vi "PI Close GPIB.vi"(0 "System no.":i32=1 min=1 max=4 step=1, 5 "error in":errorcluster) -> (14 "Was connected?":bool, 19 "error out":errorcluster)   [LabVIEW 2011]
doc: "This VI checks if the connection to the selected system is already open and, if it is, it closes this connection. \n\nValid for C-843, C-843.PM, C-844, C-865, E-710 (but must be present in Communication.llb for all other systems, too)"
uses:
  <userlib>/E710_GCS_LabVIEW/Low Level/Communication.llb/Global1.vi
panel:
  # "This vi checks if the connection to the selected system\nis already open and, if it is, it closes this connection."
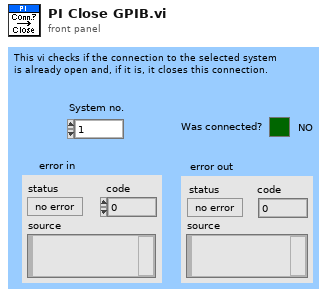
[diagram p1: front panel]
types:
  T1 = cluster{"DLL for Device":u16, "DLL Interface":u16, "Parameter":string}[]
  T2 = cluster{"RS232 Portnumber":u16, "Timeout":u32, "RS232 Baud rate":u32, "Interface":u16, "GPIB Bus":i32, "GPIB Address":i32, "GPIB Mode":i32}[]
  T3 = cluster{"RS232 Portnumber":u16, "Timeout":u32, "RS232 Baud rate":u32, "Interface":u16, "GPIB Bus":i32, "GPIB Address":i32, "GPIB Mode":i32}
  T4 = cluster{"DLL for Device":u16, "DLL Interface":u16, "Parameter":string}
  T5 = enum16{"C844_IsDLLAvailable", "C844_ConnectRS232", "C844_ConnectNIgpib", "C844_IsConnected", "C844_CloseConnection", "C844_GcsCommandset", "C844_GetError", "C844_GcsGetAnswerSize", "C844_GcsGetAnswer"}
  T6 = enum16{"C844_IsDLLAvailable", "C844_ConnectRS232", "C844_ConnectNIgpib", "C844_IsConnected", "C844_CloseConnection", "C844_GcsCommandset", "C844_GetError", "C844_GcsGetAnswerSize", "C844_GcsGetAnswer", "C843_IsDLLAvailable", "C843_Connect", "C843_IsConnected", "C843_CloseConnection", "C843_GcsCommandset", "C843_GetError", "C843_GcsGetAnswerSize", "C843_GcsGetAnswer", "E710_IsDLLAvailable", "E710_ConnectRS232", "E710_ConnectNIgpib", "E710_IsConnected", "E710_CloseConnection", "E710_GcsCommandset", "E710_GetError", "E710_GcsGetAnswerSize", "E710_GcsGetAnswer"}
  T7 = enum16{"C844_IsDLLAvailable", "C844_ConnectRS232", "C844_ConnectNIgpib", "C844_IsConnected", "C844_CloseConnection", "C844_GcsCommandset", "C844_GetError", "C844_GcsGetAnswerSize", "C844_GcsGetAnswer", "C843_IsDLLAvailable", "C843_Connect", "C843_IsConnected", "C843_CloseConnection", "C843_GcsCommandset", "C843_GetError", "C843_GcsGetAnswerSize", "C843_GcsGetAnswer", "E710_IsDLLAvailable", "E710_ConnectRS232", "E710_ConnectNIgpib", "E710_IsConnected", "E710_CloseConnection", "E710_GcsCommandset", "E710_GetError", "E710_GcsGetAnswerSize", "E710_GcsGetAnswer", "C843_PM_IsDLLAvailable", "C843_PM_Connect", "C843_PM_IsConnected", "C843_PM_CloseConnection", "C843_PM_GcsCommandset", "C843_PM_GetError", "C843_PM_GcsGetAnswerSize", "C843_PM_GcsGetAnswer", "C843_PM_GetCurrentBoardID"}
  T8 = enum16{"C844_IsDLLAvailable", "C844_ConnectRS232", "C844_ConnectNIgpib", "C844_IsConnected", "C844_CloseConnection", "C844_GcsCommandset", "C844_GetError", "C844_GcsGetAnswerSize", "C844_GcsGetAnswer", "C843_IsDLLAvailable", "C843_Connect", "C843_IsConnected", "C843_CloseConnection", "C843_GcsCommandset", "C843_GetError", "C843_GcsGetAnswerSize", "C843_GcsGetAnswer", "E710_IsDLLAvailable", "E710_ConnectRS232", "E710_ConnectNIgpib", "E710_IsConnected", "E710_CloseConnection", "E710_GcsCommandset", "E710_GetError", "E710_GcsGetAnswerSize", "E710_GcsGetAnswer", "C843_PM_IsDLLAvailable", "C843_PM_Connect", "C843_PM_IsConnected", "C843_PM_CloseConnection", "C843_PM_GcsCommandset", "C843_PM_GetError", "C843_PM_GcsGetAnswerSize", "C843_PM_GcsGetAnswer"}
  T9 = enum16{"C844_IsDLLAvailable", "C844_ConnectRS232", "C844_ConnectNIgpib", "C844_IsConnected", "C844_CloseConnection", "C844_GcsCommandset", "C844_GetError", "C844_GcsGetAnswerSize", "C844_GcsGetAnswer", "C843_IsDLLAvailable", "C843_Connect", "C843_IsConnected", "C843_CloseConnection", "C843_GcsCommandset", "C843_GetError", "C843_GcsGetAnswerSize", "C843_GcsGetAnswer", "E710_IsDLLAvailable", "E710_ConnectRS232", "E710_ConnectNIgpib", "E710_IsConnected", "E710_CloseConnection", "E710_GcsCommandset", "E710_GetError", "E710_GcsGetAnswerSize", "E710_GcsGetAnswer", "C843_PM_IsDLLAvailable", "C843_PM_Connect", "C843_PM_IsConnected", "C843_PM_CloseConnection", "C843_PM_GcsCommandset", "C843_PM_GetError", "C843_PM_GcsGetAnswerSize", "C843_PM_GcsGetAnswer", "C843_PM_GetCurrentBoardID", "C843_GetCurrentBoardID", "C865_IsDLLAvailable", "C865_ConnectRS232", "C865_IsConnected", "C865_CloseConnection", "C865_GcsCommandset", "C865_GetError", "C865_GcsGetAnswerSize", "C865_GcsGetAnswer", "C865_GetCurrentInterfaceID"}
  T10 = enum16{"C844_IsDLLAvailable", "C844_ConnectRS232", "C844_ConnectNIgpib", "C844_IsConnected", "C844_CloseConnection", "C844_GcsCommandset", "C844_GetError", "C844_GcsGetAnswerSize", "C844_GcsGetAnswer", "C843_IsDLLAvailable", "C843_Connect", "C843_IsConnected", "C843_CloseConnection", "C843_GcsCommandset", "C843_GetError", "C843_GcsGetAnswerSize", "C843_GcsGetAnswer", "E710_IsDLLAvailable", "E710_ConnectRS232", "E710_ConnectNIgpib", "E710_IsConnected", "E710_CloseConnection", "E710_GcsCommandset", "E710_GetError", "E710_GcsGetAnswerSize", "E710_GcsGetAnswer", "C843_PM_IsDLLAvailable", "C843_PM_Connect", "C843_PM_IsConnected", "C843_PM_CloseConnection", "C843_PM_GcsCommandset", "C843_PM_GetError", "C843_PM_GcsGetAnswerSize", "C843_PM_GcsGetAnswer", "C843_PM_GetCurrentBoardID", "C843_GetCurrentBoardID"}
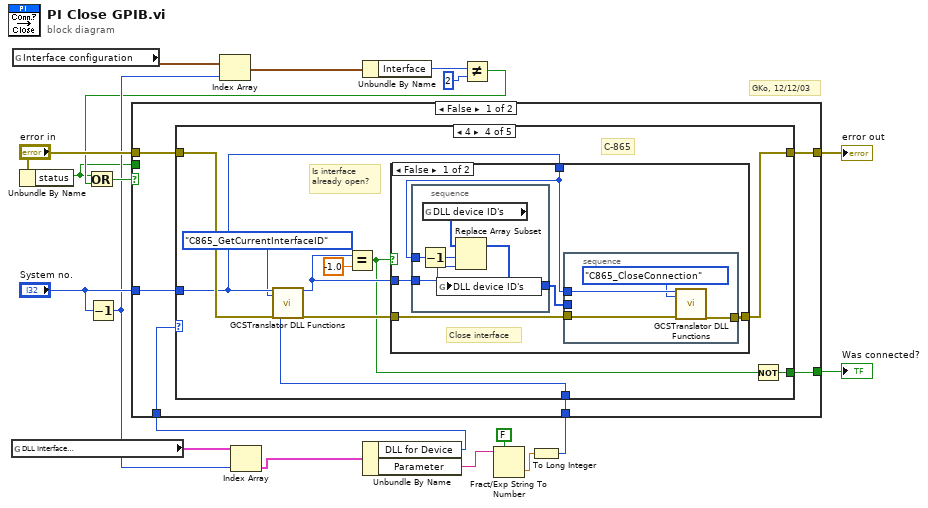
[diagram p0: block diagram]
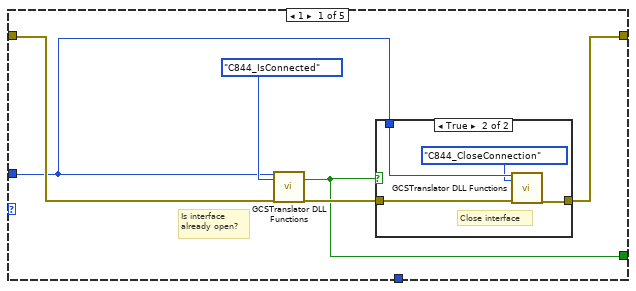
[diagram p2: hidden frame]
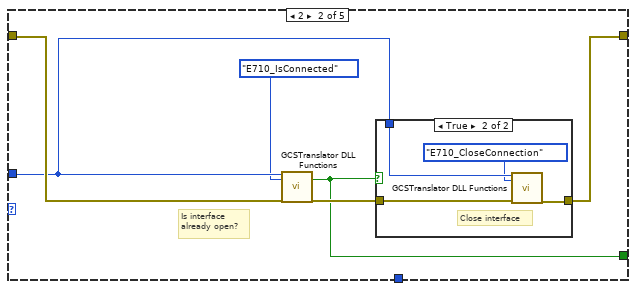
[diagram p4: hidden frame]
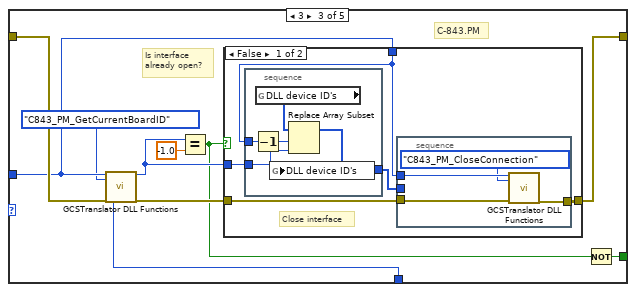
[diagram p6: hidden frame]
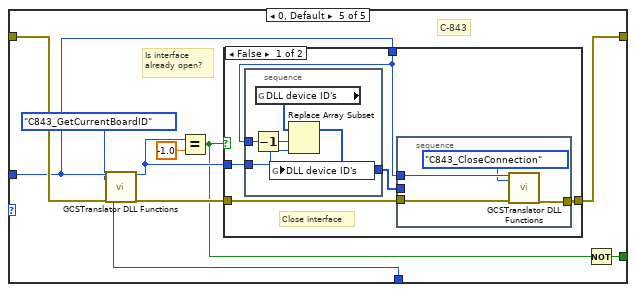
[diagram p9: hidden frame]
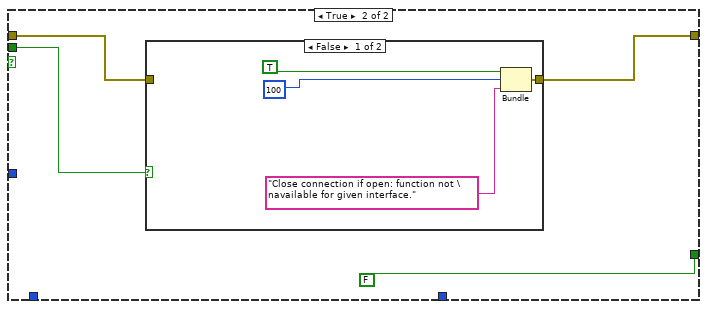
[diagram p11: hidden frame]
diagram:
  # "GKo, 12/12/03"
  n1 = global read "Global1.vi" "DLL Interface\nConfiguration"() -> (w16:T1)
  n2 = global read "Global1.vi" "Interface configuration"() -> (w13:T2)
  n3 = Unbundle By Name("error in") -> ("status"=w5:bool)
  n4 = Decrement(x="System no.") -> (x-1=w7:i32)
  n5 = Index Array(array=w13, index=w7) -> (element=w12:T3)
  n6 = Index Array(array=w16, index=w7) -> (element=w15:T4)
  n7 = Unbundle By Name(w12) -> ("Interface"=w11:u16)
  n8 = Unbundle By Name(w15) -> ("DLL for Device"=w14:u16, "Parameter"=w2:string)
  n9 = Not Equal?(x=w11, y=u16 2) -> (x != y?=w6:bool)
  n10 = Or(x=w5, y=w6) -> (x .or. y?=w9:bool)
  n11 = Fract/Exp String To Number(use system decimal point (T)=FALSE, string=w2) -> (number=w3:dbl)  [unwired: 2 in, 1 out]
  n12 = To Long Integer(number=w3) -> (32bit integer=w1:i32)
  n13 = case shown="False" w9 {
    tunnel: "System no." -> [w23 _]
    tunnel: "error in" -> [w25 w125]
    tunnel: [w24 w124] -> w18
    tunnel: [w22 FALSE ("Boolean output")] -> w17
    tunnel: w14 -> [w21 _]
    tunnel: w5 -> [_ w123]
    tunnel: w1 -> [w20 _]
    frame False {
      n14 = case shown="4" w21 {
        tunnel: w25 -> [w29 w41 w56 w81 w106]
        tunnel: [w28 w40 w55 w80 w105] -> w24
        tunnel: w23 -> [w27 w39 w54 w79 w104]
        tunnel: [w26 w38 w52 w77 w102] -> w22
        tunnel: w20 -> [_ _ w49 w74 w99]
        frame 1 {
          # "Is interface\nalready open?"
          n15 = call <userlib>:"GCSTranslator DLL Functions.vi"("System no."=w27, "Function"=T5."C844_IsConnected", "error in"=w29) -> ("Boolean output"=w26:bool, "error out"=w31:errorcluster)  [unwired: 12 in, 3 out]
          n16 = case shown="True" w26 {
            tunnel: w31 -> [w32 w36]
            tunnel: [w32 w35] -> w28
            tunnel: w27 -> [_ w34]
            frame False {
            }
            frame True {
              # "Close interface"
              n17 = call <userlib>:"GCSTranslator DLL Functions.vi"("System no."=w34, "Function"=T5."C844_CloseConnection", "error in"=w36) -> ("error out"=w35:errorcluster)  [unwired: 12 in, 4 out]
            }
          }
        }
        frame 2 {
          # "Is interface\nalready open?"
          n18 = call <userlib>:"GCSTranslator DLL Functions.vi"("System no."=w39, "Function"=T6."E710_IsConnected", "error in"=w41) -> ("Boolean output"=w38:bool, "error out"=w42:errorcluster)  [unwired: 12 in, 3 out]
          n19 = case shown="True" w38 {
            tunnel: w42 -> [w43 w47]
            tunnel: [w43 w46] -> w40
            tunnel: w39 -> [_ w45]
            frame False {
            }
            frame True {
              # "Close interface"
              n20 = call <userlib>:"GCSTranslator DLL Functions.vi"("System no."=w45, "Function"=T6."E710_CloseConnection", "error in"=w47) -> ("error out"=w46:errorcluster)  [unwired: 12 in, 4 out]
            }
          }
        }
        frame 3 {
          # "C-843.PM"
          # "Is interface\nalready open?"
          n21 = call <userlib>:"GCSTranslator DLL Functions.vi"("System no."=w54, "Function"=T7."C843_PM_GetCurrentBoardID", "error in"=w56, "Numerical input"=w49) -> ("DLL I32 Return value"=w51:i32, "error out"=w57:errorcluster)  [unwired: 11 in, 3 out]
          n22 = Equal?(x=w51, y=-1.0) -> (x = y?=w50:bool)
          n23 = case shown="False" w50 {
            tunnel: w57 -> [w62 w72]
            tunnel: [w61 w72] -> w55
            tunnel: w54 -> [w59 _]
            tunnel: w51 -> [w58 _]
            frame False {
              # "Close interface"
              n24 = stacked-sequence {
                tunnel: [w67] -> w60
                tunnel: w59 -> [w69]
                tunnel: w58 -> [w68]
                frame #0 {
                  n25 = Decrement(x=w69) -> (x-1=w70:i32)
                  n26 = global read "Global1.vi" "DLL device ID's"() -> (w71:i32[])
                  n27 = Replace Array Subset(array=w71, new element=w68, index=w70) -> (w67:i32[])
                  n28 = global write "Global1.vi" "DLL device ID's"(w67) -> ()
                }
              }
              n29 = stacked-sequence {
                tunnel: w62 -> [w66]
                tunnel: [w65] -> w61
                tunnel: w59 -> [w64]
                tunnel: w60 -> [_]
                frame #0 {
                  n30 = call <userlib>:"GCSTranslator DLL Functions.vi"("System no."=w64, "Function"=T8."C843_PM_CloseConnection", "error in"=w66) -> ("error out"=w65:errorcluster)  [unwired: 12 in, 4 out]
                }
              }
            }
            frame True {
            }
          }
          n31 = Not(x=w50) -> (.not. x?=w52:bool)
        }
        frame 4 {
          # "C-865"
          # "Is interface\nalready open?"
          n32 = call <userlib>:"GCSTranslator DLL Functions.vi"("System no."=w79, "Function"=T9."C865_GetCurrentInterfaceID", "error in"=w81, "Numerical input"=w74) -> ("DLL I32 Return value"=w76:i32, "error out"=w82:errorcluster)  [unwired: 11 in, 3 out]
          n33 = Equal?(x=w76, y=-1.0) -> (x = y?=w75:bool)
          n34 = case shown="False" w75 {
            tunnel: w82 -> [w87 w97]
            tunnel: [w86 w97] -> w80
            tunnel: w79 -> [w84 _]
            tunnel: w76 -> [w83 _]
            frame False {
              # "Close interface"
              n35 = stacked-sequence {
                tunnel: [w92] -> w85
                tunnel: w84 -> [w94]
                tunnel: w83 -> [w93]
                frame #0 {
                  n36 = Decrement(x=w94) -> (x-1=w95:i32)
                  n37 = global read "Global1.vi" "DLL device ID's"() -> (w96:i32[])
                  n38 = Replace Array Subset(array=w96, new element=w93, index=w95) -> (w92:i32[])
                  n39 = global write "Global1.vi" "DLL device ID's"(w92) -> ()
                }
              }
              n40 = stacked-sequence {
                tunnel: w87 -> [w91]
                tunnel: [w90] -> w86
                tunnel: w84 -> [w89]
                tunnel: w85 -> [_]
                frame #0 {
                  n41 = call <userlib>:"GCSTranslator DLL Functions.vi"("System no."=w89, "Function"=T9."C865_CloseConnection", "error in"=w91) -> ("error out"=w90:errorcluster)  [unwired: 12 in, 4 out]
                }
              }
            }
            frame True {
            }
          }
          n42 = Not(x=w75) -> (.not. x?=w77:bool)
        }
        frame 0, Default {
          # "C-843"
          # "Is interface\nalready open?"
          n43 = call <userlib>:"GCSTranslator DLL Functions.vi"("System no."=w104, "Function"=T10."C843_GetCurrentBoardID", "error in"=w106, "Numerical input"=w99) -> ("DLL I32 Return value"=w101:i32, "error out"=w107:errorcluster)  [unwired: 11 in, 3 out]
          n44 = Equal?(x=w101, y=-1.0) -> (x = y?=w100:bool)
          n45 = case shown="False" w100 {
            tunnel: w107 -> [w112 w122]
            tunnel: [w111 w122] -> w105
            tunnel: w104 -> [w109 _]
            tunnel: w101 -> [w108 _]
            frame False {
              # "Close interface"
              n46 = stacked-sequence {
                tunnel: [w117] -> w110
                tunnel: w109 -> [w119]
                tunnel: w108 -> [w118]
                frame #0 {
                  n47 = Decrement(x=w119) -> (x-1=w120:i32)
                  n48 = global read "Global1.vi" "DLL device ID's"() -> (w121:i32[])
                  n49 = Replace Array Subset(array=w121, new element=w118, index=w120) -> (w117:i32[])
                  n50 = global write "Global1.vi" "DLL device ID's"(w117) -> ()
                }
              }
              n51 = stacked-sequence {
                tunnel: w112 -> [w116]
                tunnel: [w115] -> w111
                tunnel: w109 -> [w114]
                tunnel: w110 -> [_]
                frame #0 {
                  n52 = call <userlib>:"GCSTranslator DLL Functions.vi"("System no."=w114, "Function"=T8."C843_CloseConnection", "error in"=w116) -> ("error out"=w115:errorcluster)  [unwired: 12 in, 4 out]
                }
              }
            }
            frame True {
            }
          }
          n53 = Not(x=w100) -> (.not. x?=w102:bool)
        }
      }
    }
    frame True {
      n54 = case shown="False" w123 {
        tunnel: [w127 w131] -> w124
        tunnel: w125 -> [_ w131]
        frame False {
          n55 = Bundle("status"=TRUE, "code"=100, "source"="Close connection if open: function not \navailable for given interface.") -> (w127:errorcluster)  [unwired: 1 in]
        }
        frame True {
        }
      }
    }
  }
  "error out" <- w18
  "Was connected?" <- w17
